vi "Get Methods by Specific Class ID.vi"(8 "error in (no error)":errorcluster, 11 "Class ID":string) -> (0 "error out":errorcluster, 3 "Methods[]":T1(array[cluster]))   [LabVIEW 2023]
doc: "<b> </b> <b> </b>\n© 2017 Q Software Innovations, LLC\nwritten by Quentin \"Q\" Alldredge\nproduced in LabVIEW 2015\n\nsupport@qsoftwareinnovations.com\nwww.qsoftwareinnovations.com\n\nAll rights reserved.\n\nRedistribution and use in source and binary forms, with or without modification, are permitted provided that the following conditions are met:\n\n * Redistributions of source code must retain the above copyright notice, this list of conditions and the following disclaimer.\n * Redistributions in binary form must reproduce the above copyright notice, this list of conditions and the following disclaimer in the documentation and/or other materials provided with the distribution.\n * Neither the name of Q Software Innovations, LLC. nor the names of its contributors may be used to endorse or promote products derived from this software without specific prior written permission.\n\nTHIS SOFTWARE IS PROVIDED BY THE COPYRIGHT HOLDERS AND CONTRIBUTORS \"AS IS\" AND ANY EXPRESS OR IMPLIED WARRANTIES, INCLUDING, BUT NOT LIMITED TO, THE IMPLIED WARRANTIES OF MERCHANTABILITY AND FITNESS FOR A PARTICULAR PURPOSE ARE DISCLAIMED. IN NO EVENT SHALL THE COPYRIGHT OWNER OR CONTRIBUTORS BE LIABLE FOR ANY DIRECT, INDIRECT, INCIDENTAL, SPECIAL, EXEMPLARY, OR CONSEQUENTIAL DAMAGES (INCLUDING, BUT NOT LIMITED TO, PROCUREMENT OF SUBSTITUTE GOODS OR SERVICES; LOSS OF USE, DATA, OR PROFITS; OR BUSINESS INTERRUPTION) HOWEVER CAUSED AND ON ANY THEORY OF LIABILITY, WHETHER IN CONTRACT, STRICT LIABILITY, OR TORT (INCLUDING NEGLIGENCE OR OTHERWISE) ARISING IN ANY WAY OUT OF THE USE OF THIS SOFTWARE, EVEN IF ADVISED OF THE POSSIBILITY OF SUCH DAMAGE."
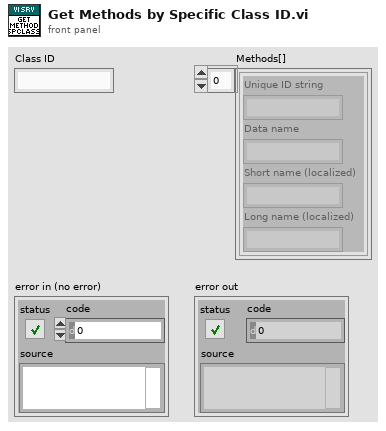
[diagram p1: front panel]
types:
  T1 = cluster{"Unique ID string":string, "Data name":string, "Short name (localized)":string, "Long name (localized)":string}[]
  T2 = cluster{"Class Name":string, "Method Info":cluster{"Unique ID string":string, "Data name":string, "Short name (localized)":string, "Long name (localized)":string}}[]
  T3 = cluster{"Unique ID string":string, "Parent ID string":string, "Class Name (unlocalized)":string, "Class Name (localized)":string}
  T4 = cluster{"Unique ID string":string, "Data name":string, "Short name (localized)":string, "Long name (localized)":string}
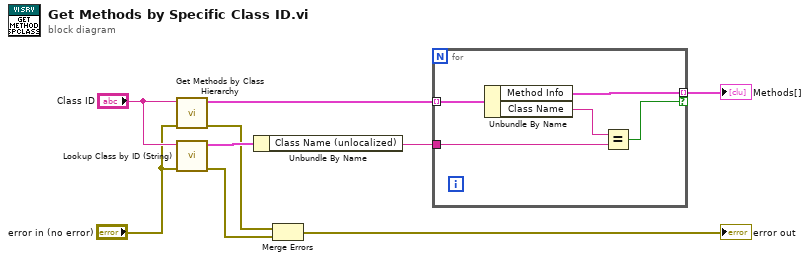
[diagram p0: block diagram]
diagram:
  n1 = call "Get Methods by Class Hierarchy.vi"("error in (no error)"="error in (no error)", "Class ID"="Class ID") -> ("error out"=w3:errorcluster, "Methods by Class Hierarchy"=w9:T2)  [unwired: 8 in]
  n2 = call "Lookup Class by ID (String).vi"("error in (no error)"="error in (no error)", "Class ID"="Class ID") -> ("error out"=w2:errorcluster, "Class Information"=w6:T3)  [unwired: 7 in, 1 out]
  n3 = Unbundle By Name(w6) -> ("Class Name (unlocalized)"=w5:string)
  n4 = Merge Errors(w3, w2) -> (→"error out":errorcluster)
  n5 = for {
    tunnel: w9 -> [w14] mode=indexing
    tunnel: w5 -> [w13]
    tunnel: [w12] -> w8 mode=indexing if=w11
    n6 = Unbundle By Name(w14) -> ("Method Info"=w12:T4, "Class Name"=w10:string)
    n7 = Equal?(x=w10, y=w13) -> (x = y?=w11:bool)
  }
  "Methods[]" <- w8
